vi "SetValue.vi"(8 "error in":errorcluster, 10 "Value":string, 11 "ProcessFullName in":refnum<class "ProcessFullName.lvclass">) -> (0 "error out":errorcluster, 3 "ProcessFullName out":refnum<class "ProcessFullName.lvclass">)   [LabVIEW 2021, in "ProligentXMLGenerator.lvlib" / "ProcessFullName.lvclass"]
uses:
  ProcessFullName.lvclass
  ProcessFullName.lvclass/ProcessFullName.ctl
  <vilib>/regexp/Match Regular Expression.xnode
  NonEmptyString/NonEmptyString.lvclass
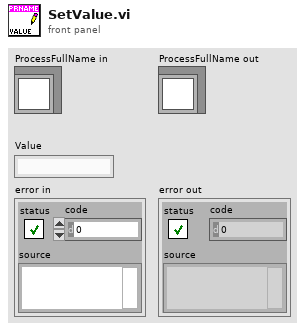
[diagram p1: front panel]
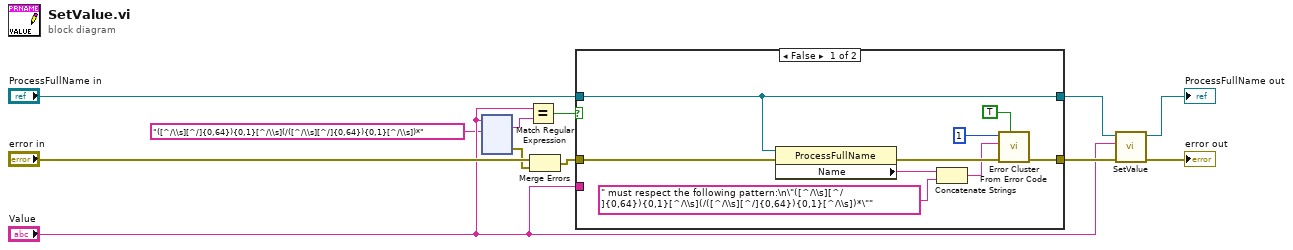
[diagram p0: block diagram]
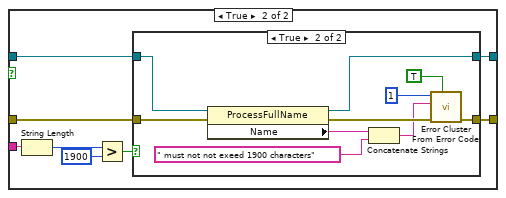
[diagram p2: hidden frame]
diagram:
  n1 = xnode ("Match Regular Expression")("input string"="Value", "regular expression"="([^/\\s][^/]{0,64}){0,1}[^/\\s](/([^/\\s][^/]{0,64}){0,1}[^/\\s])*") -> ("whole match"=w6:string, "error out"=w3:errorcluster)  [unwired: 4 in, 3 out]
  n2 = Equal?(x="Value", y=w6) -> (x = y?=w1:bool)
  n3 = Merge Errors("error in", w3) -> (w4:errorcluster)
  n4 = case shown="False" w1 {
    tunnel: "ProcessFullName in" -> [w13 w29]
    tunnel: [w14 w26] -> w8
    tunnel: [w13 w24] -> w7
    tunnel: "Value" -> [_ w23]
    tunnel: w4 -> [w15 w22]
    frame False {
      n5 = property on="Property Node" class="ProcessFullName"(reference=w13, error in=w15) -> (error out=w20:errorcluster, "Name"=w21:string)  [unwired: 1 out]
      n6 = Concatenate Strings(w21, " must respect the following pattern:\n\"([^/\\s][^/]{0,64}){0,1}[^/\\s](/([^/\\s][^/]{0,64}){0,1}[^/\\s])*\"" ("string")) -> (w19:string)
      n7 = call <vilib>:"Error Cluster From Error Code.vi"("show call chain? (False)"=TRUE, "error in (no error)"=w20, "error message (\"\")"=w19, "error code (0)"=1) -> ("error out"=w14:errorcluster)  [unwired: 5 in]
    }
    frame True {
      n8 = String Length(string=w23) -> (length=w28:i32)
      n9 = Greater?(x=w28, y=1900) -> (0:w25:bool)
      n10 = case shown="True" w25 {
        tunnel: w22 -> [w31 w36]
        tunnel: [w31 w41] -> w26
        tunnel: [w30 w34] -> w24
        tunnel: w29 -> [w30 w37]
        frame False {
        }
        frame True {
          n11 = property on="Property Node" class="ProcessFullName"(reference=w37, error in=w36) -> (reference out=w34:refnum<class "ProcessFullName.lvclass">, error out=w35:errorcluster, "Name"=w38:string)
          n12 = Concatenate Strings(w38, " must not not exeed 1900 characters" ("string")) -> (w33:string)
          n13 = call <vilib>:"Error Cluster From Error Code.vi"("show call chain? (False)"=TRUE, "error in (no error)"=w35, "error message (\"\")"=w33, "error code (0)"=1) -> ("error out"=w41:errorcluster)  [unwired: 5 in]
        }
      }
    }
  }
  n14 = call-parent "SetValue.vi"("error in"=w8, "Value"="Value", "NonEmptyString in"=w7) -> ("error out"=→"error out":errorcluster, "NonEmptyString out"=→"ProcessFullName out":refnum<class "ProcessFullName.lvclass">)  [unwired: 7 in]
